vi "query_vectorsearch.vi"(0 "vector_weviate in":refnum<class "vector_weviate.lvclass">, 5 "collection_name":string, 7 "vector":dbl[](array[numeric]), 9 "limit":u32, 11 "error in (no error)":errorcluster) -> (4 "vector_weviate out":refnum<class "vector_weviate.lvclass">, 6 "results":T1[](array[typedef]), 15 "error out":errorcluster)   [LabVIEW 2020, in "vector_weviate.lvclass"]
uses:
  vector_weviate.lvclass
  abstract_vector_base/search result.ctl
  abstract_vector_base/vector.ctl
  abstract_vector_base/abstract_vector_base.lvclass
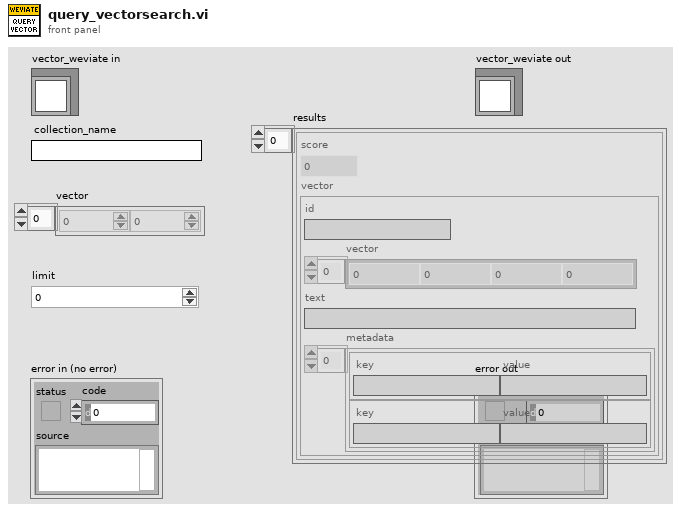
[diagram p1: front panel]
types:
  T1 = typedef "abstract_vector_base.lvclass/search result.ctl" = cluster{"score":dbl, "vector":T2}
  T2 = typedef "abstract_vector_base.lvclass/vector.ctl" = cluster{"id":string, "vector":dbl[], "text":string, "metadata":cluster{"key":string, "value":string}[]}
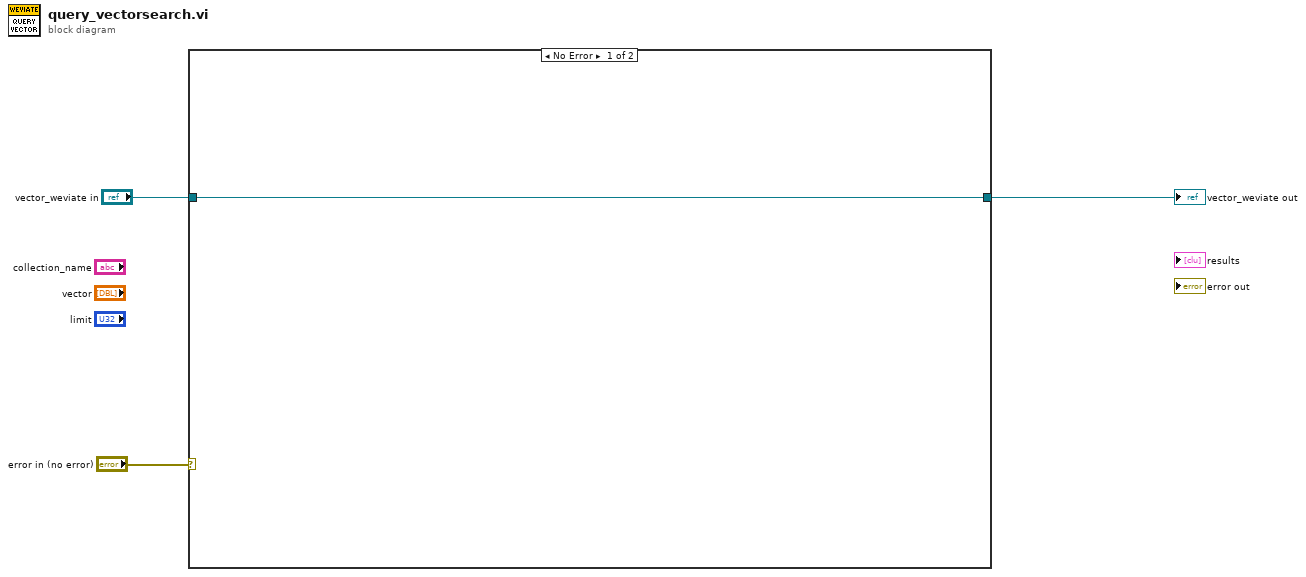
[diagram p0: block diagram]
diagram:
  n1 = case shown="No Error" "error in (no error)" {
    tunnel: "vector_weviate in" -> [w4 w5]
    tunnel: [w4 w5] -> w1
    frame No Error {
    }
    frame Error {
    }
  }
  "vector_weviate out" <- w1
